vi "p1.vi"() -> ()   [LabVIEW 2023, in "d25.lvlib"]
uses:
  d25.lvlib
  <vilib>/Utility/miscctls.llb/LVMapReplaceAction.ctl
  AOC/AOC.lvlib
panel:
  out "Answer":i32
  in  "Example":string="jqt: rhn xhk nvd\nrsh: frs pzl lsr\nxhk: hfx\ncmg: qnr nvd lhk bvb\nrhn: xhk bvb hfx\nbvb: xhk hfx\npzl: lsr hfx nvd\nqnr: nvd\nntq: jqt hfx bvb xhk\nnvd: lhk\nlsr: lhk\nrzs: qnr cmg lsr rsh\nfrs: qnr lhk lsr"
  in  "Example":bool
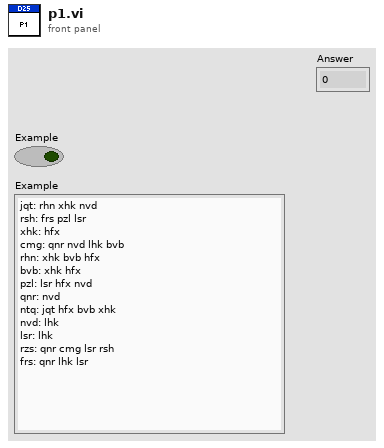
[diagram p1: front panel]
types:
  T1 = typedef "LVMapReplaceAction.ctl" = enum32{"Modify Entry only if found", "Add or Modify Entry", "Delete Entry"}
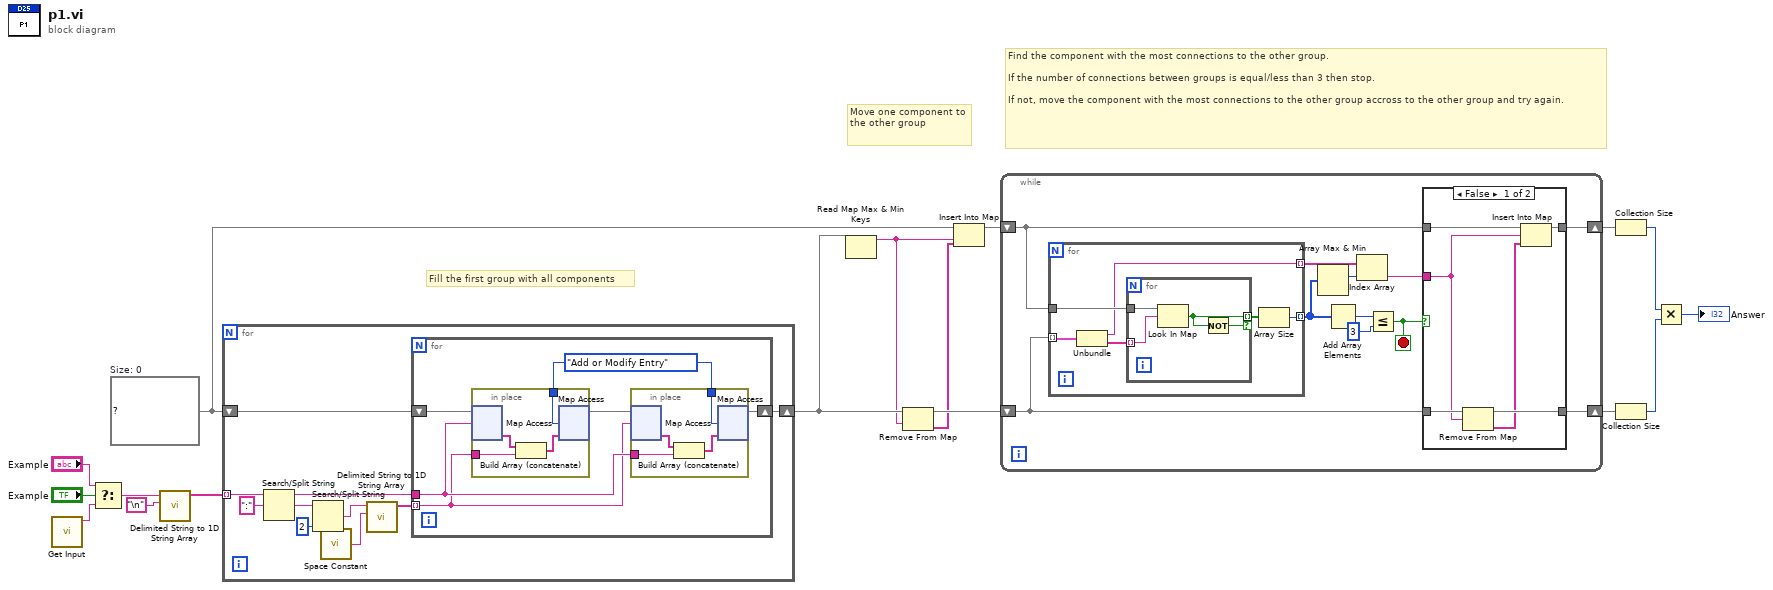
[diagram p0: block diagram]
diagram:
  w8 = map{string, string[]} {}  # Size: 0
  # "Find the component with the most connections to the other group.\n\nIf the number of connections between groups is equal/less than 3 then stop.\n\nIf not, move the component with the most connections to the other group accross to the other group and try again."
  # "Fill the first group with all components"
  # "Move one component to the other group"
  n1 = call "Get Input.vi"() -> ("Input"=w17:string)  [unwired: 11 in]
  n2 = Select(t="Example", s="Example", f=w17) -> (s? t:f=w16:string)
  n3 = call <vilib>:"Delimited String to 1D String Array.vi"("delimiter"="\n", "delimited string"=w16) -> ("string array"=w12:string[])  [unwired: 9 in]
  n4 = for {
    tunnel: w12 -> [w26] mode=indexing
    shift-right: [w23] -> w11
    shift-left: w8 -> [w27]
    n5 = Search/Split String(string=w26, search string/char (-)=":") -> (substring before match=w24:string, match + rest of string=w20:string)  [unwired: 1 in, 1 out]
    n6 = Search/Split String(string=w20, offset (0)=2) -> (match + rest of string=w19:string)  [unwired: 1 in, 2 out]
    n7 = call <vilib>:"Space Constant.vi"() -> ("String"=w21:string)
    n8 = call <vilib>:"Delimited String to 1D String Array.vi"("delimiter"=w21, "delimited string"=w19) -> ("string array"=w22:string[])  [unwired: 9 in]
    n9 = for {
      shift-right: [w31] -> w23
      shift-left: w27 -> [w33]
      tunnel: w24 -> [w30]
      tunnel: w22 -> [w29] mode=indexing
      w28 = LVMapReplaceAction."Add or Modify Entry" ("action")
      n10 = in-place {
        in-place-border: w29 -> [w41]
        in-place-border: w28 -> [w39]
        n11 = in-place-map #1(w33, w30) -> (w40:string[])  [unwired: 1 in, 1 out]
        n12 = Build Array (concatenate)(w40, w41) -> (w38:string[])
        n13 = in-place-map #1(w38, w39) -> (w32:map{string, string[]})  [unwired: 2 out]
      }
      n14 = in-place {
        in-place-border: w30 -> [w37]
        in-place-border: w28 -> [w36]
        n15 = in-place-map #2(w32, w29) -> (w35:string[])  [unwired: 1 in, 1 out]
        n16 = Build Array (concatenate)(w35, w37) -> (w34:string[])
        n17 = in-place-map #2(w34, w36) -> (w31:map{string, string[]})  [unwired: 2 out]
      }
    }
  }
  n18 = Read Map Max & Min Keys(11:w11) -> (3:w7:string)  [unwired: 1 out]
  n19 = Remove From Map(10:w7, 11:w11) -> (1:w6:string[], 3:w9:map{string, string[]})  [unwired: 1 out]
  n20 = Insert Into Map(map in=w8, key=w7, value=w6) -> (map out=w10:map{string, string[]})  [unwired: 2 out]
  n21 = while {
    shift-right: [w48] -> w5
    shift-left: w10 -> [w47]
    shift-right: [w50] -> w4
    shift-left: w9 -> [w49]
    stop <- w42 stop-if-true
    n22 = for {
      tunnel: w49 -> [w66] mode=indexing
      tunnel: w47 -> [w65]
      tunnel: [w62] -> w45 mode=indexing
      tunnel: [w61] -> w52 mode=indexing
      n23 = Unbundle(w66) -> (w61:string, w64:string[])
      n24 = for {
        tunnel: w65 -> [w70]
        tunnel: w64 -> [w69] mode=indexing
        tunnel: [w68] -> w63 mode=indexing if=w67
        n25 = Look In Map(map=w70, key=w69) -> (key not found?=w68:bool)  [unwired: 1 in, 1 out]
        n26 = Not(x=w68) -> (.not. x?=w67:bool)
      }
      n27 = Array Size(array=w63) -> (size(s)=w62:i32)
    }
    n28 = Array Max & Min(array=w45) -> (max index (indices)=w51:i32)  [unwired: 3 out]
    n29 = Add Array Elements(numeric array=w45) -> (sum=w44:i32)
    n30 = Index Array(array=w52, index=w51) -> (element=w46:string)
    n31 = Less Or Equal?(x=w44, y=3 ("x")) -> (x <= y?=w42:bool)
    n32 = case shown="False" w42 {
      tunnel: [w58 w59] -> w50
      tunnel: w49 -> [w57 w59]
      tunnel: [w56 w60] -> w48
      tunnel: w47 -> [w55 w60]
      tunnel: w46 -> [w53 _]
      frame False {
        n33 = Remove From Map(10:w53, 11:w57) -> (1:w54:string[], 3:w58:map{string, string[]})  [unwired: 1 out]
        n34 = Insert Into Map(map in=w55, key=w53, value=w54) -> (map out=w56:map{string, string[]})  [unwired: 2 out]
      }
      frame True {
      }
    }
  }
  n35 = Collection Size(1:w5) -> (0:w3:i32)
  n36 = Collection Size(1:w4) -> (0:w2:i32)
  n37 = Multiply(x=w3, y=w2) -> (x*y=→"Answer":i32)
